vi "Centrifuge Pause Selection.vi"(8 "error in (no error)":errorcluster, 11 "Pump Settings In":T1={"Output Device"=enum."Default", "EPOS4 Settings"={"VISA resource name"="", "axis"={"keyHandle"=1, "nodeId"=1}, "Simulated?"=FALSE}}) -> (0 "error out":errorcluster, 1 "Connection Error":bool, 3 "Pump Settings Out":T1={"Output Device"=enum."Default", "EPOS4 Settings"={"VISA resource name"="", "axis"={"keyHandle"=1, "nodeId"=1}, "Simulated?"=FALSE}})   [LabVIEW 2018, in "Centrifuge Module.lvlib" / "Centrifuge Module Engine.lvlib"]
uses:
  Centrifuge Module Engine.lvlib
  Centrifuge Settings Cluster.ctl
  EPOS4/Controls/Device Selection.ctl
  EPOS4/Controls/EPOS Communication Settings.ctl
  Centrifuge Module.lvlib
  EPOS4/EPOS4.lvlib
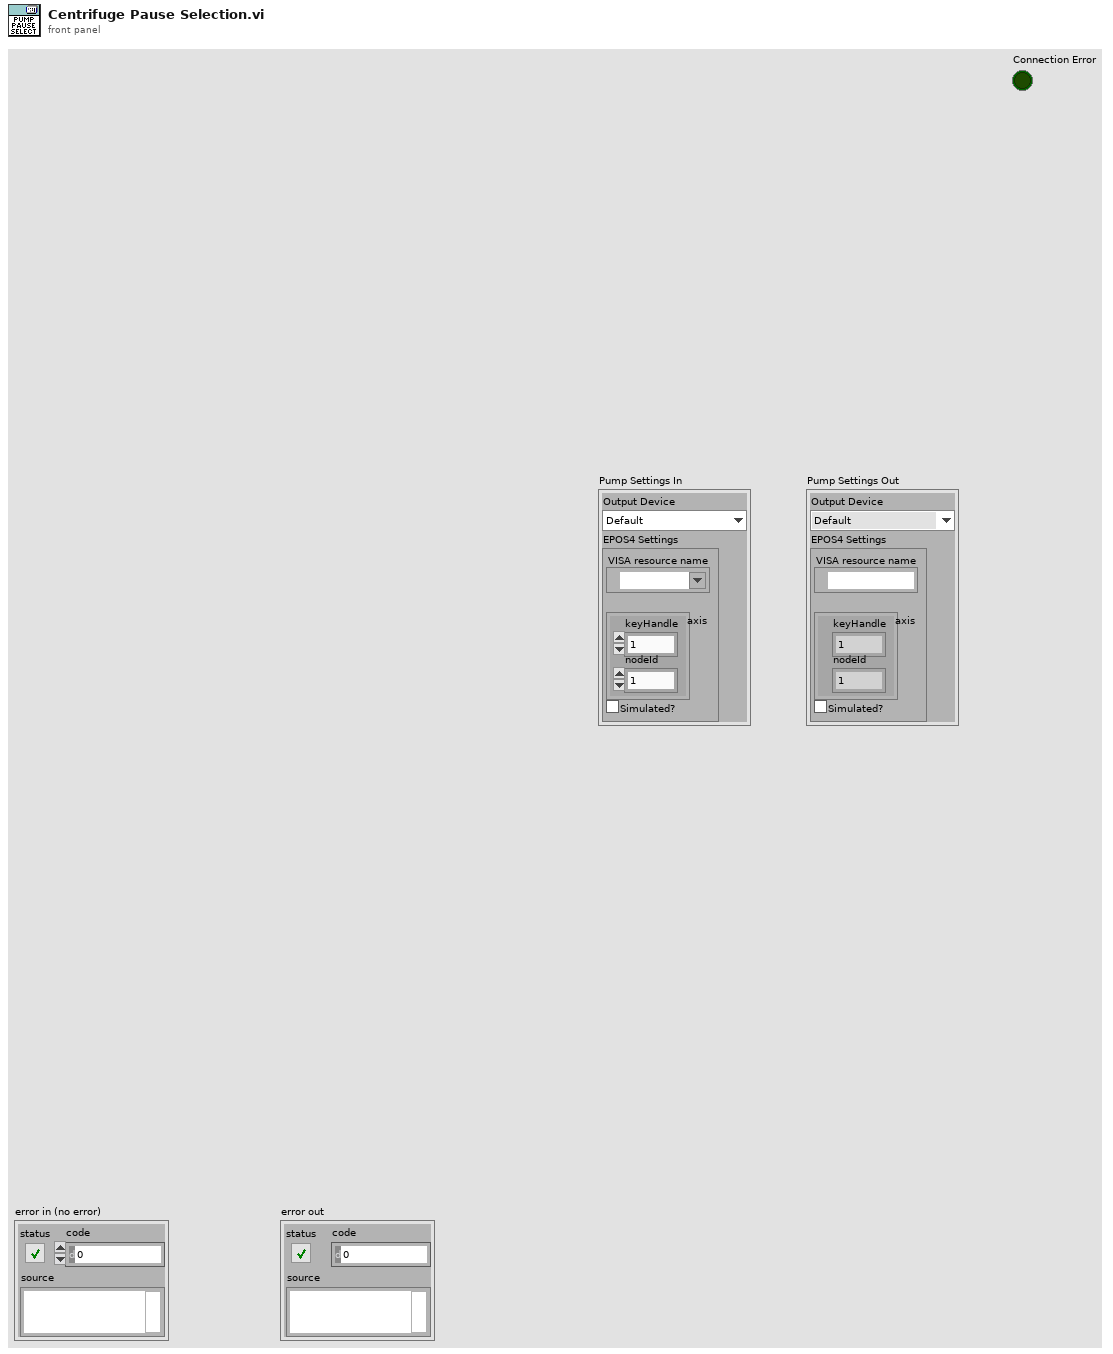
[diagram p1: front panel]
types:
  T1 = typedef "Centrifuge Module.lvlib/Centrifuge Settings Cluster.ctl" = cluster{"Output Device":T2, "EPOS4 Settings":T3}
  T2 = typedef "Device Selection.ctl" = enum16{"Default", "EPOS4"}
  T3 = typedef "EPOS4.lvlib/EPOS Communication Settings.ctl" = cluster{"VISA resource name":refnum<visa-resource-name>, "axis":cluster{"keyHandle":u32, "nodeId":u16}, "Simulated?":bool}
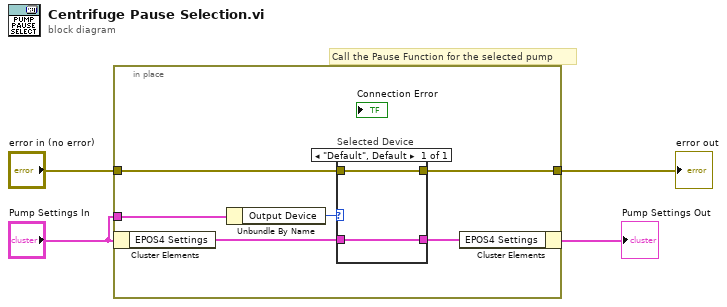
[diagram p0: block diagram]
diagram:
  # "Call the Pause Function for the selected pump"
  n1 = in-place {
    in-place-border: "error in (no error)" -> [w10]
    in-place-border: [w9] -> w3
    in-place-border: "Pump Settings In" -> [w6]
    n2 = in-place-cluster #1("Pump Settings In") -> ("EPOS4 Settings"=w8:T3)
    n3 = Unbundle By Name(w6) -> ("Output Device"=w5:T2)
    n4 = case "Selected Device" shown="\"Default\", Default" w5 {
      tunnel: w8 -> [w12]
      tunnel: [w12] -> w7
      tunnel: [w11] -> w9
      tunnel: w10 -> [w11]
      frame "Default", Default {
      }
    }
    n5 = in-place-cluster #1("EPOS4 Settings"=w7) -> (→"Pump Settings Out":T1)
  }
  "error out" <- w3
